vi "Time-Delayed Send Message Core.vi"(6 "Message Priority (Normal)":T1=enum."Normal", 7 "How Many Copies (0 = infinite repeat)":u32, 8 "Time To Wait":i32=1000, 9 "Delivery Notifier":refnum<notifier>, 10 "Message":refnum<class "Message.lvclass">, 11 "Message Enqueuer":refnum<class "Message Enqueuer.lvclass">) -> ()   [LabVIEW 2013]
doc: "This VI forms the core processing loop for the time-delayed messages. This VI may be called directly if the desired behavior is for the caller to wait until the messages have been sent before continuing, but the usual usage of this VI is to call <b>Time-Delayed Send Message.vi</b> which will launch an asynch clone of this VI so that the caller can proceed with other work instead of waiting for the time out. \n\nSee Context Help for <b>Time-Delayed Send Message.vi</b> for further details."
uses:
  <vilib>/ActorFramework/Message Enqueuer/Message Enqueuer.lvclass
  <vilib>/ActorFramework/Message/Message.lvclass
  <vilib>/ActorFramework/Time-Delayed Send Message/Time-Delay Override Options.ctl
  <vilib>/ActorFramework/Message Enqueuer/Message Priority.ctl
  <vilib>/ActorFramework/Message Enqueuer/Message Enqueuer.lvclass/Message Enqueuer.ctl
  <vilib>/ActorFramework/Message Priority Queue/Priority Enqueue.vi
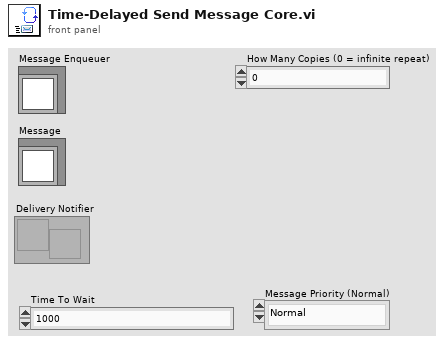
[diagram p1: front panel]
types:
  T1 = typedef "Actor Framework.lvlib/Message Enqueuer.lvclass/Message Priority.ctl" = enum16{"Low", "Normal", "High"}
  T2 = typedef "Time-Delay Override Options.ctl" = enum16{"Send next copy now", "Skip next scheduled copy", "Send next copy now and stop all further copies", "Stop all further copies"}
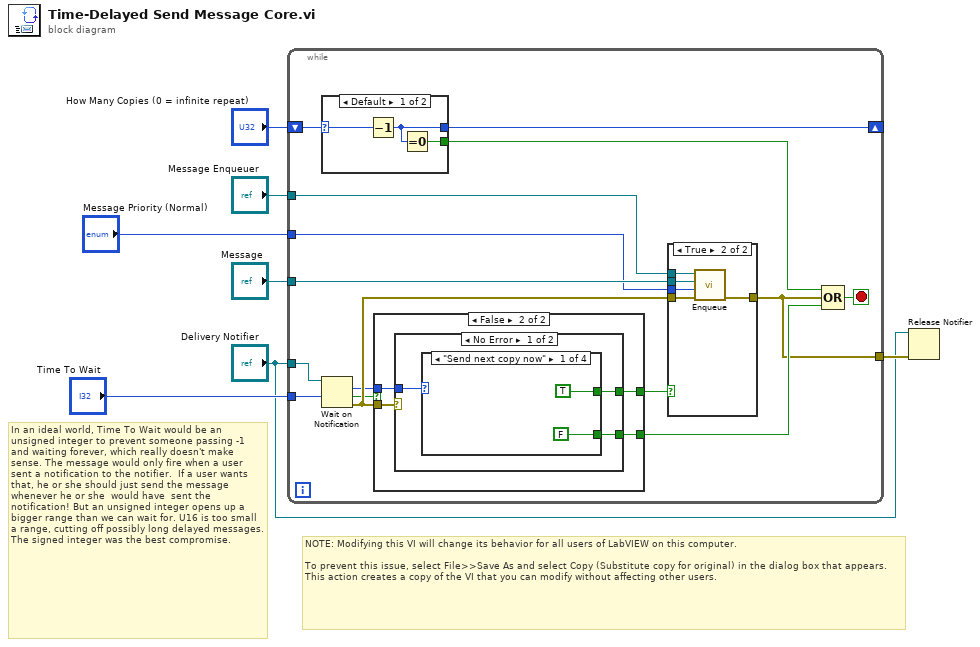
[diagram p0: block diagram]
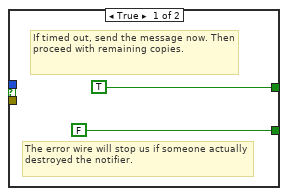
[diagram p2: hidden frame]
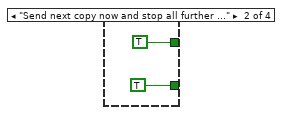
[diagram p3: hidden frame]
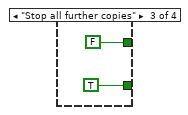
[diagram p4: hidden frame]
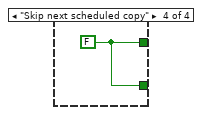
[diagram p5: hidden frame]
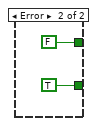
[diagram p6: hidden frame]
diagram:
  # "NOTE: Modifying this VI will change its behavior for all users of LabVIEW on this computer.\n\nTo prevent this issue, select File>>Save As and select Copy (Substitute copy for original) in the dialog box that appears. This action creates a copy of the VI that you can modify without affecting other users."
  # "In an ideal world, Time To Wait would be an unsigned integer to prevent someone passing -1 and waiting forever, which really doesn't make sense. The message would only fire when a user sent a notification to the notifier.  If a user wants that, he or she should just send the message whenever he or she  would have  sent the notification! But an unsigned integer opens up a bigger range than we can wait for. U16 is too small a range, cutting off possibly long delayed messages. The signed integer was the best compromise."
  n1 = while {
    shift-right: [w20] -> _
    shift-left: "How Many Copies (0 = infinite repeat)" -> [w21]
    tunnel: "Delivery Notifier" -> [w19]
    tunnel: "Message Enqueuer" -> [w18]
    tunnel: "Message" -> [w17]
    tunnel: "Time To Wait" -> [w11]
    tunnel: [w9] -> w3
    tunnel: "Message Priority (Normal)" -> [w8]
    stop <- w16 stop-if-true
    n2 = case shown="Default" w21 {
      selector: w21 -> [w49 w50]
      tunnel: [w48 w50] -> w20
      tunnel: [w47 _] -> w15
      frame Default {
        n3 = Decrement(x=w49) -> (x-1=w48:u32)
        n4 = Equal To 0?(x=w48) -> (x = 0?=w47:bool)
      }
      frame 0 {
      }
    }
    n5 = Wait on Notification(notifier=w19, timeout in ms (-1)=w11) -> (notification=w12:T2, timed out?=w14:bool, error out=w22:errorcluster)  [unwired: 2 in, 1 out]
    n6 = case shown="False" w14 {
      tunnel: [TRUE w27] -> w13
      tunnel: w12 -> [_ w26]
      tunnel: w22 -> [_ w28]
      tunnel: [FALSE w25] -> w10
      frame True {
        # "The error wire will stop us if someone actually destroyed the notifier."
        # "If timed out, send the message now. Then proceed with remaining copies."
      }
      frame False {
        n7 = case shown="No Error" w28 {
          tunnel: [w30 FALSE] -> w27
          tunnel: w26 -> [w31 _]
          tunnel: [w29 TRUE] -> w25
          frame No Error {
            n8 = case shown="\"Send next copy now\"" w31 {
              tunnel: [TRUE TRUE FALSE w38] -> w30
              tunnel: [FALSE TRUE TRUE w38] -> w29
              frame "Send next copy now" {
              }
              frame "Send next copy now and stop all further copies" {
              }
              frame "Stop all further copies" {
              }
              frame "Skip next scheduled copy" {
                w38 = FALSE
              }
            }
          }
          frame Error {
          }
        }
      }
    }
    n9 = case shown="True" w13 {
      tunnel: w18 -> [_ w46]
      tunnel: w17 -> [_ w45]
      tunnel: w22 -> [w41 w44]
      tunnel: [w41 w43] -> w9
      tunnel: w8 -> [_ w42]
      frame False {
      }
      frame True {
        n10 = call <vilib>:"Enqueue.vi"("error in (no error)"=w44, "Message Priority (Normal)"=w42, "Message"=w45, "Message Enqueuer in"=w46) -> ("error out"=w43:errorcluster)  [unwired: 6 in, 1 out]
      }
    }
    n11 = Compound Arithmetic op=OR(w15, w9, w10) -> (w16:bool)
  }
  n12 = Release Notifier(notifier="Delivery Notifier", error in (no error)=w3) -> ()  [unwired: 1 in, 3 out]
